vi "CMI ADS127L21 - Get Measured Reference Freq.vi"(8 "error in (no error)":errorcluster, 11 "session in":T1 {"channels"."Channel" min=1 max=8 step=1; "channels"."Range [Vpk]" items=["±1.65V", "±2V"]}) -> (0 "error out":errorcluster, 2 "freq [Hz]":dbl, 3 "session out":T1 {"channels"."Channel" min=1 max=8 step=1; "channels"."Range [Vpk]" items=["±1.65V", "±2V"]})   [LabVIEW 2020]
doc: "Get measured frequency of selected reference clock."
uses:
  CMI ADS127L21 - Session.ctl
  CMI ADS127L21 - Record Channel.ctl
  CMI ADS127L21 - Input Range.ctl
  CMI ADS127L21 - Input Mode.ctl
  CMI ADS127L21 - Input Impedance.ctl
  CMI ADS127L21 - EXTOUT Mode.ctl
  CMI ADS127L21 - EXTOUT Polarity.ctl
  <vilib>/Instr/_visa.llb/VISA Flush IO Buffer Mask.ctl
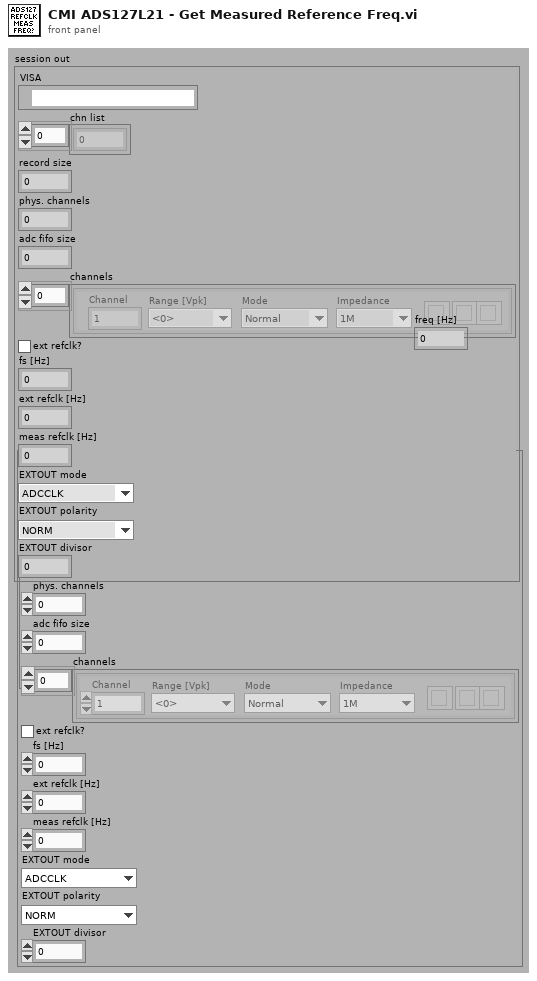
[diagram p1: front panel]
types:
  T1 = typedef "CMI ADS127L21 - Session.ctl" = cluster{"VISA":refnum<visa-resource-name>, "chn list":i32[], "record size":i32, "phys. channels":i32, "adc fifo size":i32, "channels":T2[], "ext refclk?":bool, "fs [Hz]":dbl, "ext refclk [Hz]":dbl, "meas refclk [Hz]":dbl, "EXTOUT mode":T6, "EXTOUT polarity":T7, "EXTOUT divisor":i32}
  T2 = typedef "CMI ADS127L21 - Record Channel.ctl" = cluster{"Range [Vpk]":T3, "Channel":i32, "Mode":T4, "Impedance":T5, "btn clr":bool, "btn up":bool, "btn down":bool}
  T3 = typedef "CMI ADS127L21 - Input Range.ctl" = dbl
  T4 = typedef "CMI ADS127L21 - Input Mode.ctl" = enum16{"Normal", "Inverted", "GND"}
  T5 = typedef "CMI ADS127L21 - Input Impedance.ctl" = enum16{"1M", "1k5"}
  T6 = typedef "CMI ADS127L21 - EXTOUT Mode.ctl" = enum16{"ADCCLK", "REFCLK", "SMPLCLK", "FIRST"}
  T7 = typedef "CMI ADS127L21 - EXTOUT Polarity.ctl" = enum16{"NORM", "INV"}
  T8 = typedef "VISA Flush IO Buffer Mask.ctl" = u16
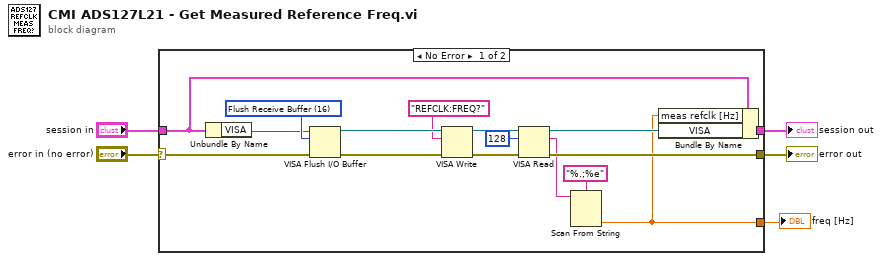
[diagram p0: block diagram]
diagram:
  n1 = case shown="No Error" "error in (no error)" {
    selector: "error in (no error)" -> [w17 w23]
    tunnel: "session in" -> [w20 w22]
    tunnel: [w21 w22] -> w4
    tunnel: [w9 w23] -> w3
    tunnel: [w6 _] -> w1
    frame No Error {
      w19 = T8 16 items=["Flush Receive Buffer"=16, "Write Transmit Buffer to Device"=32, "Flush Receive Buffer (No I/O)"=64, "Flush Transmit Buffer"=128] ("Mask")
      n2 = Unbundle By Name(w20) -> ("VISA"=w18:refnum<visa-resource-name>)
      n3 = VISA Flush I/O Buffer(VISA resource name=w18, mask (16)=w19, error in (no error)=w17) -> (VISA resource name out=w15:refnum<visa-resource-name>, error out=w16:errorcluster)
      n4 = VISA Write(VISA resource name=w15, write buffer="REFCLK:FREQ?", error in (no error)=w16) -> (VISA resource name out=w12:refnum<visa-resource-name>, error out=w13:errorcluster)  [unwired: 1 out]
      n5 = VISA Read(VISA resource name=w12, byte count=u32 128, error in (no error)=w13) -> (VISA resource name out=w11:refnum<visa-resource-name>, read buffer=w8:string, error out=w9:errorcluster)  [unwired: 1 out]
      n6 = Scan From String(format string="%.;%e", input string=w8) -> (output 1=w6:dbl)  [unwired: 3 in, 3 out]
      n7 = Bundle By Name(cluster=w20, "meas refclk [Hz]"=w6, "VISA"=w11) -> (w21:T1)
    }
    frame Error {
    }
  }
  "error out" <- w3
  "session out" <- w4
  "freq [Hz]" <- w1
